vi "Update Context for Owned Processes.vi"(8 "error in (no error)":errorcluster, 11 "Application In":refnum<class "Application.lvclass">) -> (0 "error out":errorcluster, 3 "Application Out":refnum<class "Application.lvclass">)   [LabVIEW 2020, in "Application.lvclass"]
uses:
  Application.lvclass
  C:/Users/anton/Documents/GitHub/Triarc-Framework/source/Framework/Process/Process.lvclass
  Application.lvclass/Application.ctl
  Process/Process.lvclass/Process.ctl
  Process/Public/Lifecycle/Get Lifecycle State.vi
  Process/Public/Lifecycle/Leave Process Loop.vi
  <vilib>/Utility/error.llb/Error Cluster From Error Code.vi
  Process/Process.lvclass
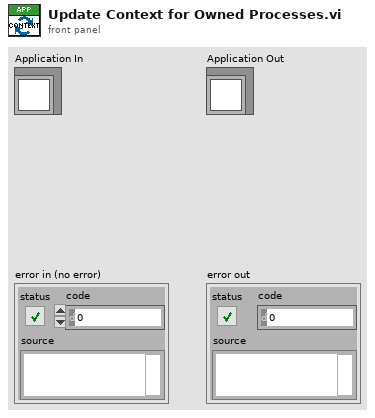
[diagram p1: front panel]
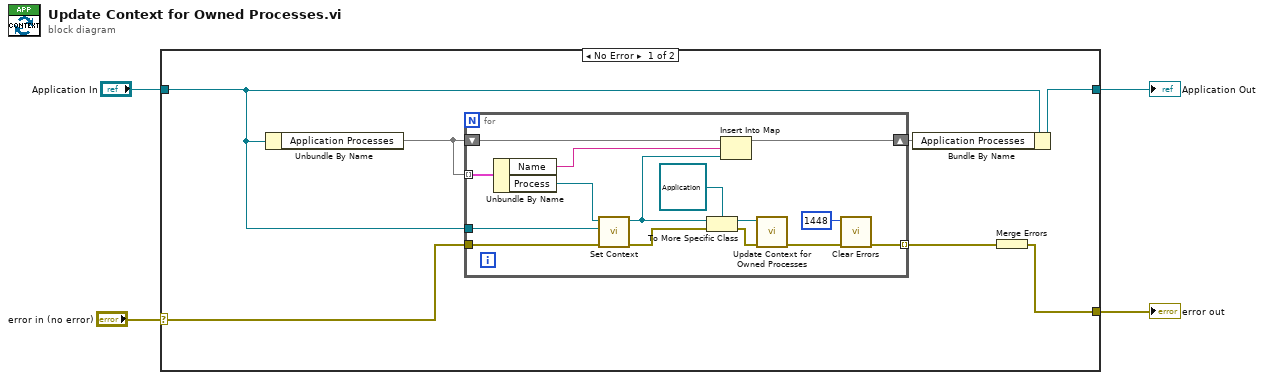
[diagram p0: block diagram]
diagram:
  n1 = case shown="No Error" "error in (no error)" {
    selector: "error in (no error)" -> [w8 w27]
    tunnel: [w11 w28] -> w4
    tunnel: [w10 w27] -> w3
    tunnel: "Application In" -> [w5 w28]
    frame No Error {
      n2 = Unbundle By Name(w5) -> ("Application Processes"=w7:map{string, refnum<class "Process.lvclass">})
      n3 = for {
        tunnel: w8 -> [w26]
        tunnel: w5 -> [w25]
        tunnel: [w14] -> w9 mode=indexing
        tunnel: w7 -> [w24] mode=indexing
        shift-right: [w20] -> w6
        shift-left: w7 -> [w22]
        n4 = Unbundle By Name(w24) -> ("Name"=w21:string, "Process"=w23:refnum<class "Process.lvclass">)
        n5 = call "Set Context.vi"("error in (no error)"=w26, "Process Context"=w25, "Process In"=w23) -> ("error out"=w19:errorcluster, "Process Out"=w12:refnum<class "Process.lvclass">)  [unwired: 7 in]
        n6 = To More Specific Class(target class=refnum<class "Application.lvclass"> refnum ("Application Out"), reference=w12, error in=w19) -> (specific class reference=w18:refnum<class "Application.lvclass">, error out=w16:errorcluster)
        n7 = Insert Into Map(map in=w22, key=w21, value=w12) -> (map out=w20:map{string, refnum<class "Process.lvclass">})  [unwired: 2 out]
        n8 = call "Update Context for Owned Processes.vi"("error in (no error)"=w16, "Application In"=w18) -> ("error out"=w15:errorcluster)  [unwired: 8 in, 1 out]
        n9 = call <vilib>:"Clear Errors.vi"("error in (no error)"=w15, "specific error code to clear (0: all)"=1448) -> ("error out"=w14:errorcluster)  [unwired: 4 in, 1 out]
      }
      n10 = Bundle By Name(cluster=w5, "Application Processes"=w6) -> (w11:refnum<class "Application.lvclass">)
      n11 = Merge Errors(w9) -> (w10:errorcluster)
    }
    frame Error {
    }
  }
  "Application Out" <- w4
  "error out" <- w3
